vi "UI_Update_timeline.vi"(0 "Timeline values in":T2, 1 "Loaded.timeline":dbl[](array[numeric]), 5 "Timeline absolute min&max in":cluster{"Tl. min":dbl, "TL. max":dbl}, 7 "Timeline absolute min&max indices in":T1, 9 "Timeline min&max in":cluster{"Tl. min":dbl, "TL. max":dbl}, 11 "Timeline min&max indices in":T1, 12 "Error In":errorcluster) -> (4 "Timeline values out":T2, 6 "Cur. pos. slider index":i32, 8 "Update timeline index?":bool, 10 "Timeline min&max out":cluster{"Tl. min":dbl, "TL. max":dbl}, 14 "Error Out":errorcluster, 15 "Timeline min&max indices out":T1)   [LabVIEW 2018, in "Tracker.lvlib"]
uses:
  Tracker.lvlib
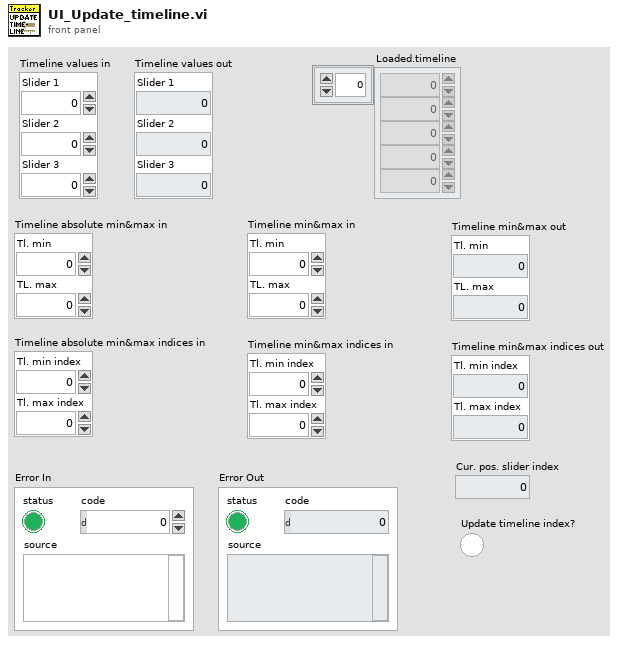
[diagram p1: front panel]
types:
  T1 = cluster{"Tl. min index":i32, "Tl. max index":i32}
  T2 = cluster{"Slider 1":dbl, "Slider 2":dbl, "Slider 3":dbl}
  T3 = cluster{"Slider 1":dbl, "Slider 2":dbl, "Slider 1":dbl}
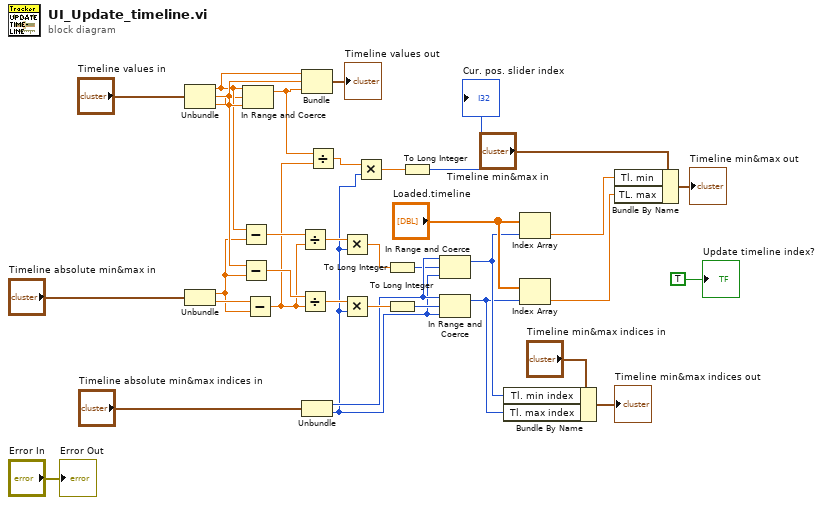
[diagram p0: block diagram]
diagram:
  n1 = Unbundle("Timeline values in") -> ("Slider 1"=w28:dbl, "Slider 2"=w32:dbl, "Slider 3"=w27:dbl)
  n2 = Unbundle("Timeline absolute min&max in") -> ("Tl. min"=w9:dbl, "TL. max"=w22:dbl)
  n3 = Subtract(x=w28, y=w9) -> (x-y=w11:dbl)
  n4 = Subtract(x=w32, y=w9) -> (x-y=w10:dbl)
  n5 = In Range and Coerce(upper limit=w28, x=w27, lower limit=w32) -> (coerced(x)=w7:dbl)  [unwired: 1 out]
  n6 = Subtract(x=w22, y=w9) -> (x-y=w6:dbl)
  n7 = Divide(x=w11, y=w6) -> (x/y=w29:dbl)
  n8 = Divide(x=w10, y=w6) -> (x/y=w34:dbl)
  n9 = Bundle("Slider 1"=w28, "Slider 2"=w32, "Slider 1"=w7) -> (→"Timeline values out":T3)  [unwired: 1 in]
  n10 = Unbundle("Timeline absolute min&max indices in") -> ("Tl. min index"=w12:i32, "Tl. max index"=w4:i32)
  n11 = Divide(x=w7, y=w6) -> (x/y=w5:dbl)
  n12 = Multiply(x=w29, y=w4) -> (x*y=w30:dbl)
  n13 = Multiply(x=w34, y=w4) -> (x*y=w33:dbl)
  n14 = Multiply(x=w5, y=w4) -> (x*y=w3:dbl)
  n15 = To Long Integer(number=w30) -> (32bit integer=w8:i32)
  n16 = To Long Integer(number=w33) -> (32bit integer=w15:i32)
  n17 = To Long Integer(number=w3) -> (32bit integer=→"Cur. pos. slider index":i32)
  n18 = In Range and Coerce(upper limit=w12, x=w8, lower limit=w4) -> (coerced(x)=w14:i32)  [unwired: 1 out]
  n19 = In Range and Coerce(upper limit=w12, x=w15, lower limit=w4) -> (coerced(x)=w13:i32)  [unwired: 1 out]
  n20 = Bundle By Name(cluster="Timeline min&max indices in", "Tl. min index"=w14, "Tl. max index"=w13) -> (→"Timeline min&max indices out":T1)
  n21 = Index Array(array="Loaded.timeline", index=w14) -> (element=w31:dbl)
  n22 = Index Array(array="Loaded.timeline", index=w13) -> (element=w35:dbl)
  n23 = Bundle By Name(cluster="Timeline min&max in", "Tl. min"=w31, "TL. max"=w35) -> (→"Timeline min&max out":cluster{"Tl. min":dbl, "TL. max":dbl})
  "Error Out" <- "Error In"
  "Update timeline index?" <- TRUE ("Update timeline index?")
